vi "LidarAntiDust (SubVI).vi"(9 "Magnitude in":dbl[](array[numeric]), 10 "BodyRange":dbl, 11 "MaxRange":dbl) -> (3 "Magnitude out":dbl[](array[numeric]))   [LabVIEW 2012]
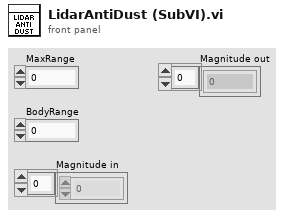
[diagram p1: front panel]
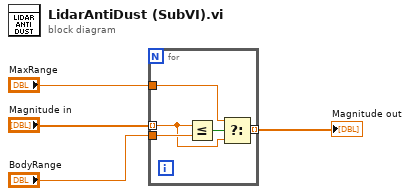
[diagram p0: block diagram]
diagram:
  n1 = for {
    tunnel: "Magnitude in" -> [w5] mode=indexing
    tunnel: "BodyRange" -> [w8]
    tunnel: "MaxRange" -> [w7]
    tunnel: [w6] -> w4 mode=indexing
    n2 = Less Or Equal?(x=w5, y=w8) -> (x <= y?=w9:bool)
    n3 = Select(t=w7, s=w9, f=w5) -> (s? t:f=w6:dbl)
  }
  "Magnitude out" <- w4
